vi "get description.vi"(8 "error in (no error)":errorcluster, 11 "Task in":refnum<class "Task.lvclass">) -> (0 "error out":errorcluster, 1 "Task summary":string, 2 "Task description":string, 3 "Task out":refnum<class "Task.lvclass">)   [LabVIEW 2020, in "Tasks.lvlib" / "Task.lvclass"]
uses:
  Task.lvclass
  Task.lvclass/Task.ctl
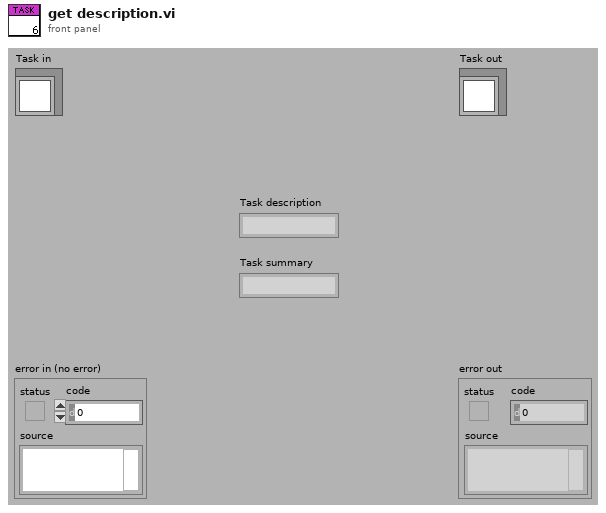
[diagram p1: front panel]
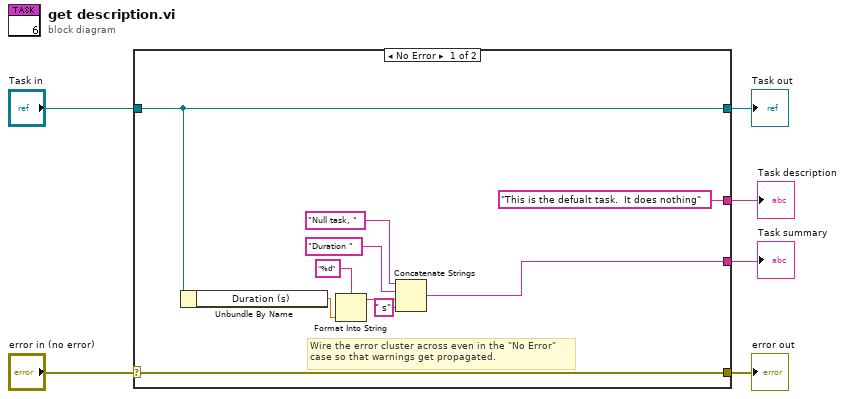
[diagram p0: block diagram]
diagram:
  n1 = case shown="No Error" "error in (no error)" {
    selector: "error in (no error)" -> [w16 w18]
    tunnel: [w16 w18] -> w5
    tunnel: [w7 w17] -> w3
    tunnel: "Task in" -> [w7 w17]
    tunnel: [w8 _] -> w2
    tunnel: ["This is the defualt task.  It does nothing" ("Task description") _] -> w1
    frame No Error {
      # "Wire the error cluster across even in the \"No Error\"\ncase so that warnings get propagated."
      n2 = Unbundle By Name(w7) -> ("Duration (s)"=w14:dbl)
      n3 = Format Into String(format string="%d", w14) -> (resulting string=w12:string)  [unwired: 2 in, 1 out]
      n4 = Concatenate Strings("Null task, " ("Task summary"), "Duration " ("initial string"), w12, " s" ("string")) -> (w8:string)
    }
    frame Error {
    }
  }
  "error out" <- w5
  "Task out" <- w3
  "Task description" <- w1
  "Task summary" <- w2
